vi "Timer_StateMachine_Simple_Example.vi"() -> ()   [LabVIEW 2019]
uses:
  <vilib>/Utility/semaphor.llb/Obtain Semaphore Reference.vi
  <vilib>/Rock Robotics/WPI/ThirdParty/JAS_Junk/TrajLib/Trajectory_Library.lvlib
panel:
  in  "Tab Control":enum32{"Control Panel"}(tab)
  out "Sequence\nRunning":bool
  in  "Start \nSequence":bool
  out "Trend":cluster{"CurrentTImer":dbl, dbl, dbl, dbl}(graph)
  out "Action 1":bool
  in  "Stop \nSequence":bool
  out "Action 2":bool
  out "State":i32
  # "Timer - Simple State Machine - Example"
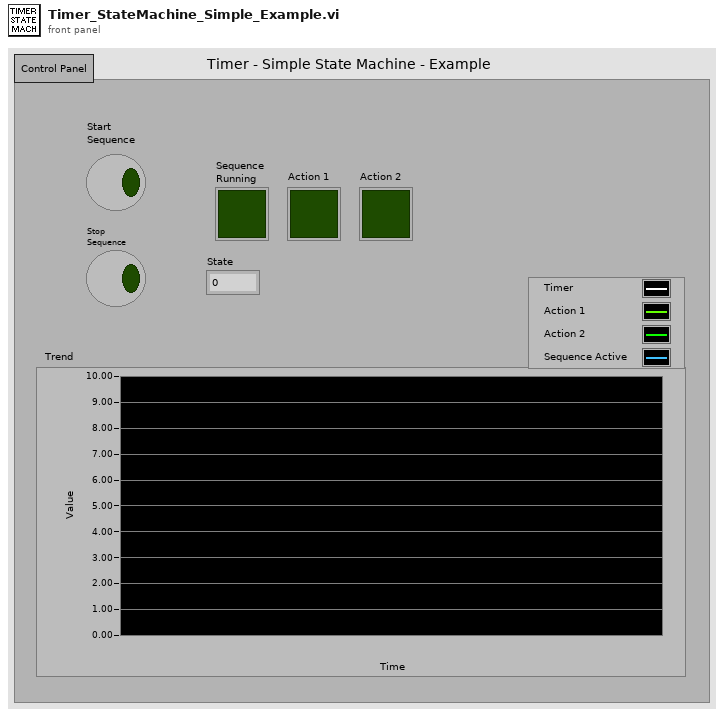
[diagram p1: front panel]
types:
  T1 = typedef "Trajectory_Library.lvlib/TIMER.ctl" = cluster{"StartTime":dbl, "Accumulated TIme":dbl, "Running":bool, "semaphore":T2}
  T2 = typedef "Semaphore RefNum" = refnum<k1>
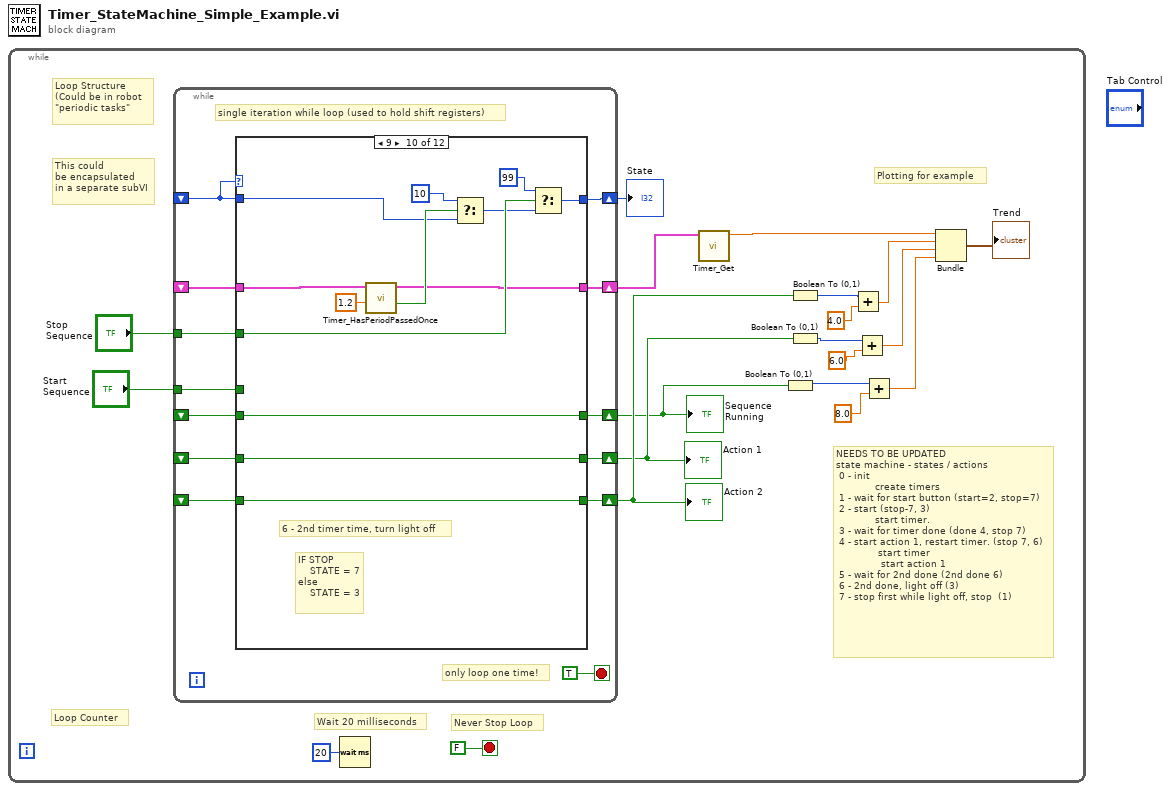
[diagram p0: block diagram]
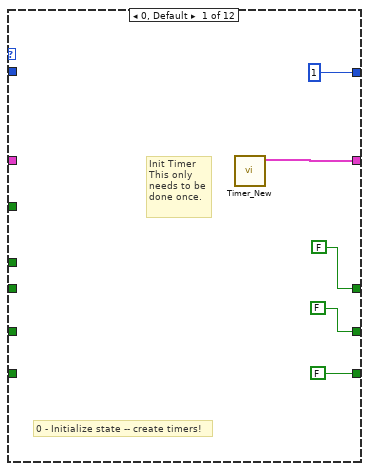
[diagram p2: hidden frame]
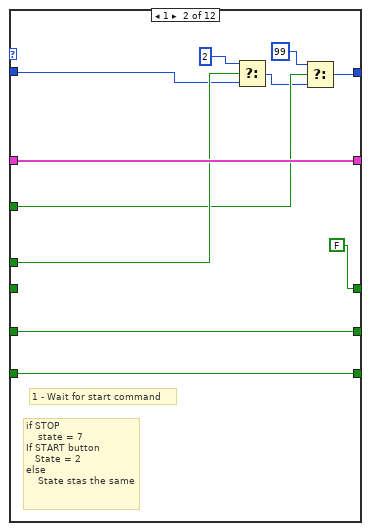
[diagram p3: hidden frame]
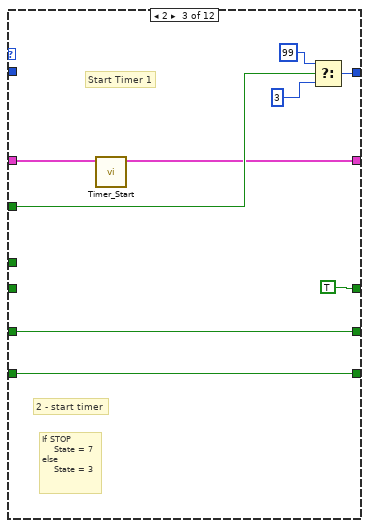
[diagram p4: hidden frame]
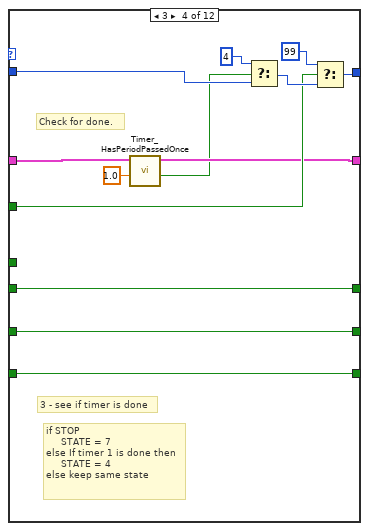
[diagram p5: hidden frame]
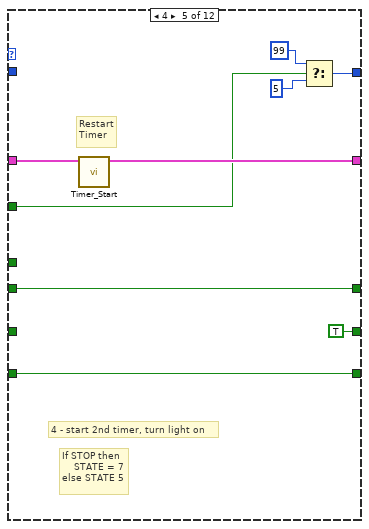
[diagram p6: hidden frame]
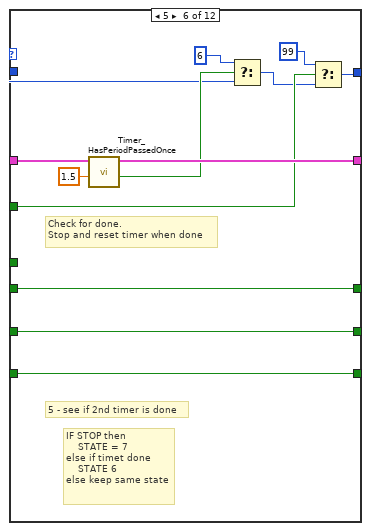
[diagram p7: hidden frame]
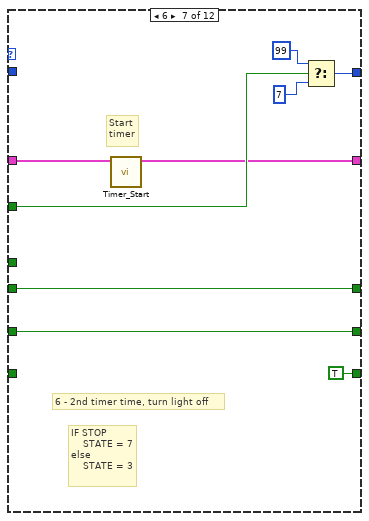
[diagram p8: hidden frame]
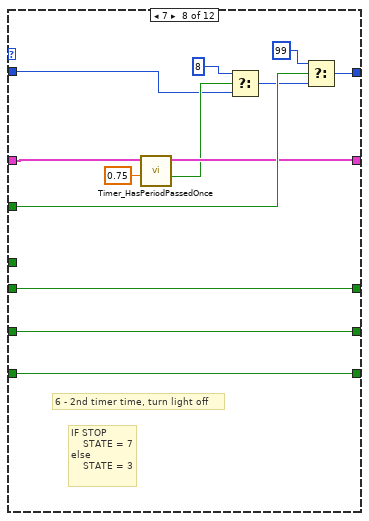
[diagram p9: hidden frame]
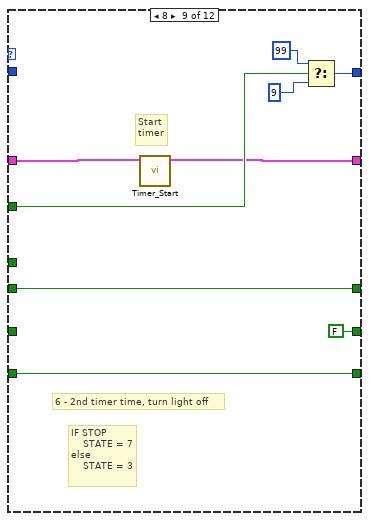
[diagram p10: hidden frame]
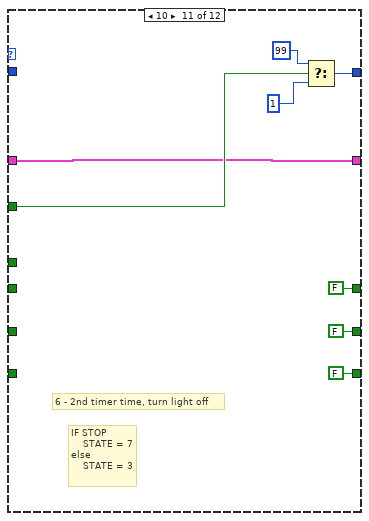
[diagram p11: hidden frame]
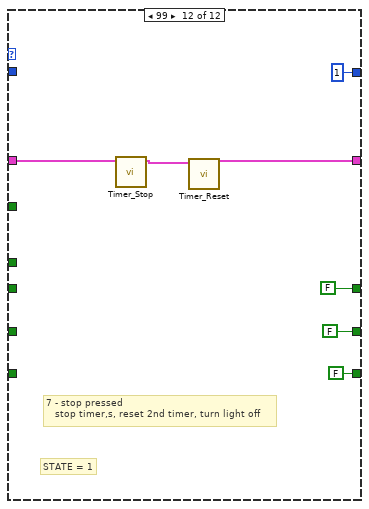
[diagram p12: hidden frame]
diagram:
  n1 = while {
    stop <- FALSE stop-if-true
    # "Plotting for example"
    # "This could\nbe encapsulated\nin a separate subVI"
    # "Loop Structure\n(Could be in robot\n\"periodic tasks\""
    # "NEEDS TO BE UPDATED\nstate machine - states / actions\n 0 - init \n             create timers\n 1 - wait for start button (start=2, stop=7)\n 2 - start (stop-7, 3)\n             start timer.\n 3 - wait for timer done (done 4, stop 7)\n 4 - start action 1, restart timer. (stop 7, 6)\n              start timer\n               start action 1\n 5 - wait for 2nd done (2nd done 6)\n 6 - 2nd done, light off (3)\n 7 - stop first while light off, stop  (1)"
    # "Loop Counter"
    # "Never Stop Loop"
    # "Wait 20 milliseconds"
    n2 = while {
      shift-right: [w31] -> w18
      shift-left: _ -> [w29]
      shift-right: [w32] -> w16
      shift-left: _ -> [w28]
      tunnel: "Start \nSequence" -> [w30]
      shift-right: [w27] -> w11
      shift-left: _ -> [w26]
      tunnel: "Stop \nSequence" -> [w25]
      shift-right: [w24] -> w12
      shift-left: _ -> [w23]
      shift-right: [w22] -> w10
      shift-left: _ -> [w21]
      stop <- TRUE stop-if-true
      # "only loop one time!"
      # "single iteration while loop (used to hold shift registers)"
      n3 = case shown="9" w29 {
        tunnel: [w38 w49 w51 w62 w79 w90 w94 w108 w116 w128 w142 w149] -> w32
        tunnel: [1 w41 w54 w65 w77 w85 w100 w114 w123 w136 w144 1 ("t")] -> w31
        tunnel: w30 -> [_ w48 _ _ _ _ _ _ _ _ _ _]
        tunnel: w29 -> [_ w47 _ w70 _ w87 _ w103 _ w127 _ _]
        tunnel: w28 -> [_ w49 w52 w63 w80 w91 w95 w109 w117 w129 w142 w151]
        tunnel: [FALSE w45 w58 w69 TRUE w93 w97 w112 FALSE w125 FALSE FALSE] -> w27
        tunnel: w26 -> [_ w45 w58 w69 _ w93 w97 w112 _ w125 _ _]
        tunnel: w25 -> [_ w43 w55 w66 w75 w84 w99 w113 w122 w135 w143 _]
        tunnel: [FALSE w40 w53 w59 w74 w81 TRUE w107 w120 w133 FALSE FALSE] -> w24
        tunnel: w23 -> [_ w40 w53 w59 w74 w81 _ w107 w120 w133 _ _]
        tunnel: [FALSE FALSE TRUE w60 w72 w82 w96 w111 w121 w134 FALSE FALSE] -> w22
        tunnel: w21 -> [_ _ _ w60 w72 w82 w96 w111 w121 w134 _ _]
        frame 0, Default {
          # "0 - Initialize state -- create timers!"
          # "Init Timer\nThis only\nneeds to be\ndone once."
          n4 = call <vilib>:"Timer_New.vi"() -> ("TIMER"=w38:T1)  [unwired: 11 in]
        }
        frame 1 {
          # "if STOP \n    state = 7\nIf START button\n   State = 2\nelse\n    State stas the same"
          # "1 - Wait for start command"
          n5 = Select(t=2, s=w48, f=w47) -> (s? t:f=w42:i32)
          n6 = Select(t=99, s=w43, f=w42) -> (s? t:f=w41:i32)
        }
        frame 2 {
          # "If STOP\n    State = 7\nelse\n    State = 3"
          # "Start Timer 1"
          # "2 - start timer"
          n7 = call <vilib>:"Timer_Start.vi"("in Timer"=w52) -> ("out Timer"=w51:T1)  [unwired: 10 in]
          n8 = Select(t=99, s=w55, f=3) -> (s? t:f=w54:i32)
        }
        frame 3 {
          # "if STOP \n     STATE = 7\nelse If timer 1 is done then\n     STATE = 4\nelse keep same state"
          # "Check for done."
          # "3 - see if timer is done"
          n9 = call <vilib>:"Timer_HasPeriodPassedOnce.vi"("Period"=1.0, "in Timer"=w63) -> ("Expired"=w61:bool, "out Timer"=w62:T1)  [unwired: 7 in, 1 out]
          n10 = Select(t=4, s=w61, f=w70) -> (s? t:f=w67:i32)
          n11 = Select(t=99, s=w66, f=w67) -> (s? t:f=w65:i32)
        }
        frame 4 {
          # "Restart\nTimer"
          # "If STOP then\n    STATE = 7\nelse STATE 5"
          # "4 - start 2nd timer, turn light on"
          n12 = call <vilib>:"Timer_Start.vi"("in Timer"=w80) -> ("out Timer"=w79:T1)  [unwired: 10 in]
          n13 = Select(t=99, s=w75, f=5 ("t")) -> (s? t:f=w77:i32)
        }
        frame 5 {
          # "IF STOP then\n    STATE = 7\nelse if timet done\n    STATE 6\nelse keep same state"
          # "Check for done.\nStop and reset timer when done"
          # "5 - see if 2nd timer is done"
          n14 = call <vilib>:"Timer_HasPeriodPassedOnce.vi"("Period"=1.5, "in Timer"=w91) -> ("Expired"=w88:bool, "out Timer"=w90:T1)  [unwired: 7 in, 1 out]
          n15 = Select(t=6, s=w88, f=w87) -> (s? t:f=w83:i32)
          n16 = Select(t=99, s=w84, f=w83) -> (s? t:f=w85:i32)
        }
        frame 6 {
          # "Start\ntimer"
          # "IF STOP\n    STATE = 7\nelse\n    STATE = 3"
          # "6 - 2nd timer time, turn light off"
          n17 = call <vilib>:"Timer_Start.vi"("in Timer"=w95) -> ("out Timer"=w94:T1)  [unwired: 10 in]
          n18 = Select(t=99, s=w99, f=7 ("t")) -> (s? t:f=w100:i32)
        }
        frame 7 {
          # "IF STOP\n    STATE = 7\nelse\n    STATE = 3"
          # "6 - 2nd timer time, turn light off"
          n19 = call <vilib>:"Timer_HasPeriodPassedOnce.vi"("Period"=0.75, "in Timer"=w109) -> ("Expired"=w104:bool, "out Timer"=w108:T1)  [unwired: 7 in, 1 out]
          n20 = Select(t=8, s=w104, f=w103) -> (s? t:f=w105:i32)
          n21 = Select(t=99, s=w113, f=w105) -> (s? t:f=w114:i32)
        }
        frame 8 {
          # "Start\ntimer"
          # "IF STOP\n    STATE = 7\nelse\n    STATE = 3"
          # "6 - 2nd timer time, turn light off"
          n22 = call <vilib>:"Timer_Start.vi"("in Timer"=w117) -> ("out Timer"=w116:T1)  [unwired: 10 in]
          n23 = Select(t=99, s=w122, f=9 ("t")) -> (s? t:f=w123:i32)
        }
        frame 9 {
          # "IF STOP\n    STATE = 7\nelse\n    STATE = 3"
          # "6 - 2nd timer time, turn light off"
          n24 = call <vilib>:"Timer_HasPeriodPassedOnce.vi"("Period"=1.2, "in Timer"=w129) -> ("Expired"=w130:bool, "out Timer"=w128:T1)  [unwired: 7 in, 1 out]
          n25 = Select(t=10, s=w130, f=w127) -> (s? t:f=w126:i32)
          n26 = Select(t=99, s=w135, f=w126) -> (s? t:f=w136:i32)
        }
        frame 10 {
          # "IF STOP\n    STATE = 7\nelse\n    STATE = 3"
          # "6 - 2nd timer time, turn light off"
          n27 = Select(t=99, s=w143, f=1) -> (s? t:f=w144:i32)
        }
        frame 99 {
          # "STATE = 1"
          # "7 - stop pressed\n   stop timer,s, reset 2nd timer, turn light off"
          n28 = call <vilib>:"Timer_Stop.vi"("in Timer"=w151) -> ("out Timer"=w150:T1)  [unwired: 10 in]
          n29 = call <vilib>:"Timer_Reset.vi"("in TIMER"=w150) -> ("out TIMER"=w149:T1)  [unwired: 10 in]
        }
      }
    }
    "Action 1" <- w11
    "State" <- w18
    "Action 2" <- w12
    "Sequence\nRunning" <- w10
    n30 = Wait (ms)(milliseconds to wait=u32 20) -> ()  [unwired: 1 out]
    n31 = call <vilib>:"Timer_Get.vi"("TIMER"=w16) -> ("CurrentTImer"=w13:dbl)  [unwired: 10 in]
    n32 = Boolean To (0,1)(Boolean=w10) -> (0, 1=w2:i16)
    n33 = Boolean To (0,1)(Boolean=w12) -> (0, 1=w8:i16)
    n34 = Boolean To (0,1)(Boolean=w11) -> (0, 1=w5:i16)
    n35 = Add(x=w8, y=4.0) -> (x+y=w9:dbl)
    n36 = Add(x=w5, y=6.0) -> (x+y=w4:dbl)
    n37 = Add(x=w2, y=8.0) -> (x+y=w1:dbl)
    n38 = Bundle("CurrentTImer"=w13, w9, w4, w1) -> (→"Trend":cluster{"CurrentTImer":dbl, dbl, dbl, dbl})  [unwired: 1 in]
  }
